vi "Test Buffer.vi"() -> ()   [LabVIEW 2017]
uses:
  PMU Buffer/Buffer state.ctl
  PMU Buffer/Buffer Settings.ctl
  PMU Buffer/Buffer DATA cluster.ctl
  PMU Buffer/PMU data buffer.lvlib
panel:
  out "Service 2 (All Buffer)":sgl[](array[numeric])
  out "Service 1 (Last 20)":sgl[](array[numeric])
  out "Should Get: 2":dbl[](array[numeric])
  out "Service 2 (1 shot)":sgl[](array[numeric])
  out "Service 1 (1 by 1)":sgl[](array[numeric])
  out "Should Get:":dbl[](array[numeric])
  # "Tests \nTest 1: Add and retrieve elements 1 by 1 in the buffer and fill the buffer entirely:\n- Compare the concatenated output of service 1 and the full output of service 2\nTest 2: Add 1 more element:\n- Compare the output of getting the whole buffer (Service 2) and the last <buffer size> elements (service 1)"
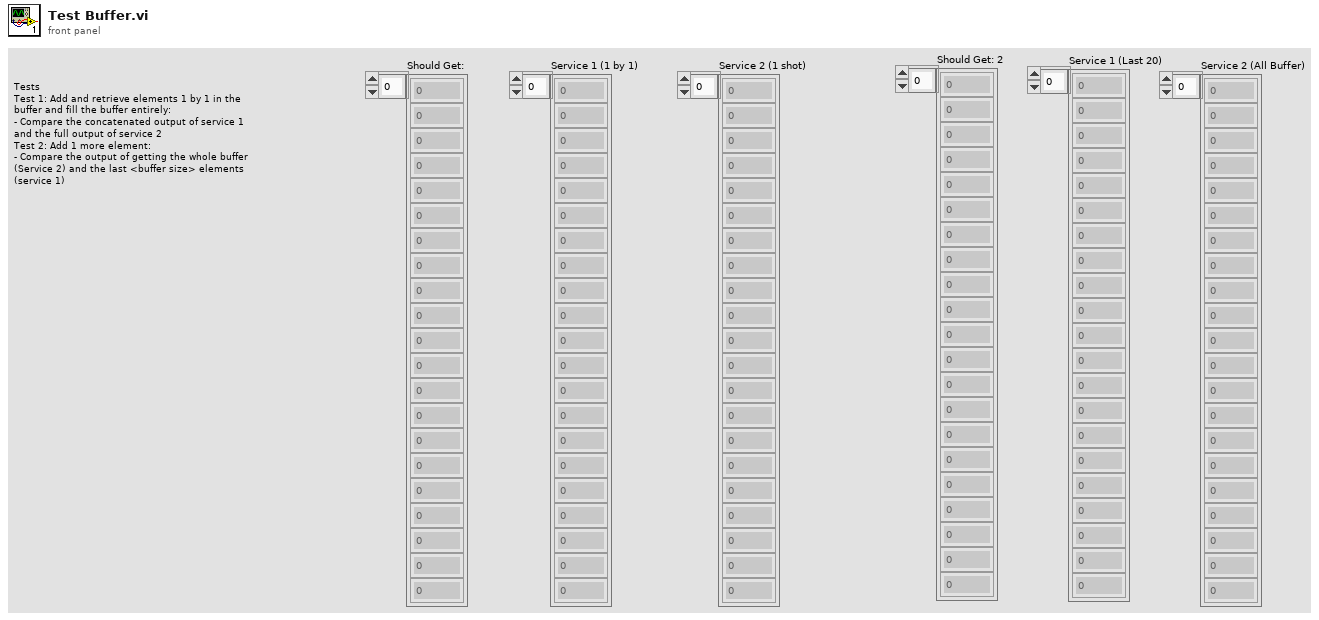
[diagram p1: front panel]
types:
  T1 = typedef "PMU data buffer.lvlib/Buffer DATA cluster.ctl" = cluster{timestamp, csg[], sgl[]}
  T2 = typedef "PMU data buffer.lvlib/Buffer state.ctl" = enum16{"Init", "Change Size", "Flush", "Exit", "Add", "Get", "Hist_Toggle", "Add_Serv"}
  T3 = typedef "PMU data buffer.lvlib/Buffer Settings.ctl" = cluster{"Index":i32, "Size":i32, "Samples":i32, "Ordered ?":bool}
  T4 = typedef "PMU data buffer.lvlib/Buffer DATA OUT ordered.ctl" = cluster{"Timestamp":timestamp[], "Phasor":csg[][], "Analog":sgl[][]}
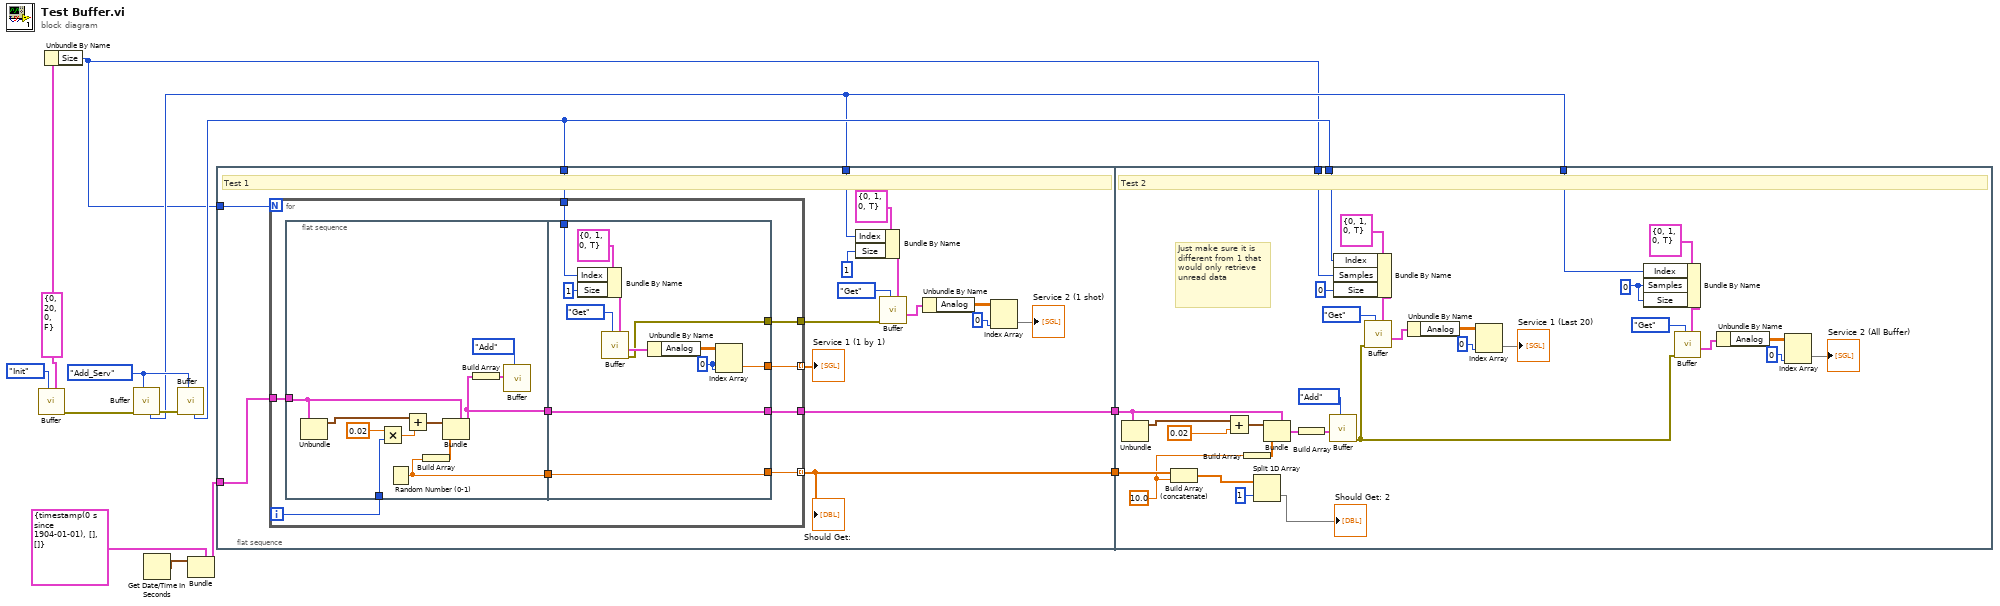
[diagram p0: block diagram]
diagram:
  w6 = Buffer_state."Add_Serv" ("Mode")
  w8 = T3 {"Index"=0, "Size"=20, "Samples"=0, "Ordered ?"=FALSE} ("Parameters")
  n1 = call "Buffer.vi"("Parameters"=w8, "Mode"=Buffer_state."Init") -> ("Error OUT"=w13:errorcluster)  [unwired: 5 in, 4 out]
  n2 = Unbundle By Name(w8) -> ("Size"=w1:i32)
  n3 = call "Buffer.vi"("Mode"=w6, "Error IN"=w13) -> ("Error OUT"=w7:errorcluster, "Index"=w2:i32)  [unwired: 5 in, 3 out]
  n4 = Get Date/Time In Seconds() -> (seconds since 1Jan1904=w9:timestamp)
  n5 = call "Buffer.vi"("Mode"=w6, "Error IN"=w7) -> ("Index"=w3:i32)  [unwired: 5 in, 4 out]
  n6 = Bundle(cluster=T1 {timestamp(0 s since 1904-01-01), [], []} ("PMU data buffer.lvlib:Buffer DATA cluster"), w9) -> (w10:T1)  [unwired: 2 in]
  n7 = flat-sequence {
    tunnel: w10 -> [w29]
    tunnel: w3 -> [w15]
    tunnel: w2 -> [w17]
    tunnel: [w19] -> w5
    tunnel: [w18] -> w4
    tunnel: w1 -> [w14]
    tunnel: w5 -> [w94]
    tunnel: w4 -> [w86]
    tunnel: w3 -> [w71]
    tunnel: w2 -> [w70]
    tunnel: w1 -> [w62]
    frame #0 {
      # "Test 1"
      n8 = for {
        N: w14 -> [_]
        tunnel: w29 -> [w38]
        tunnel: [w35] -> w19 mode=indexing
        tunnel: [w34] -> w28 mode=indexing
        tunnel: [w32] -> w18
        tunnel: [w31] -> w16
        tunnel: w15 -> [w30]
        i -> [w37]
        n9 = flat-sequence {
          tunnel: w38 -> [w47]
          tunnel: w37 -> [w43]
          tunnel: [w40] -> w36
          tunnel: [w39] -> w33
          tunnel: [w56] -> w35
          tunnel: w36 -> [w56]
          tunnel: [w53] -> w34
          tunnel: w33 -> [w52]
          tunnel: [w52] -> w32
          tunnel: [w51] -> w31
          tunnel: w30 -> [w50]
          frame #0 {
            n10 = Unbundle(w47) -> (w46:timestamp)  [unwired: 2 out]
            n11 = Multiply(x=0.02, y=w43) -> (x*y=w44:dbl)
            n12 = Random Number (0-1)() -> (number: 0 to 1=w40:dbl)
            n13 = Add(x=w46, y=w44) -> (x+y=w45:timestamp)
            n14 = Build Array(w40) -> (w41:dbl[])
            n15 = Bundle(cluster=w47, w45, w41) -> (w39:T1)  [unwired: 1 in]
            n16 = Build Array(w39) -> (w48:T1[])
            n17 = call "Buffer.vi"("Mode"=Buffer_state."Add", "DATA IN"=w48) -> ()  [unwired: 5 in, 5 out]
          }
          frame #1 {
            w54 = 0 ("index (row)")
            n18 = Bundle By Name(cluster=T3 {"Index"=0, "Size"=1, "Samples"=0, "Ordered ?"=TRUE} ("Parameters"), "Index"=w50, "Size"=1) -> (w59:T3)
            n19 = call "Buffer.vi"("Parameters"=w59, "Mode"=Buffer_state."Get") -> ("Error OUT"=w51:errorcluster, "Output"=w58:T4)  [unwired: 5 in, 3 out]
            n20 = Unbundle By Name(w58) -> ("Analog"=w55:sgl[][])
            n21 = Index Array(array=w55, index (row)=w54, index (col)=w54) -> (element=w53:sgl)
          }
        }
      }
      "Should Get:" <- w19
      "Service 1 (1 by 1)" <- w28
      n22 = Bundle By Name(cluster=T3 {"Index"=0, "Size"=1, "Samples"=0, "Ordered ?"=TRUE} ("Parameters"), "Index"=w17, "Size"=1) -> (w26:T3)
      n23 = call "Buffer.vi"("Parameters"=w26, "Mode"=Buffer_state."Get", "Error IN"=w16) -> ("Output"=w22:T4)  [unwired: 4 in, 4 out]
      n24 = Unbundle By Name(w22) -> ("Analog"=w23:sgl[][])
      n25 = Index Array(array=w23, index (col)=0 ("index (row)")) -> (element=→"Service 2 (1 shot)":sgl[])  [unwired: 1 in]
    }
    frame #1 {
      w63 = 0 ("Size")
      w90 = 10.0 ("number: 0 to 1")
      # "Just make sure it is different from 1 that would only retrieve unread data"
      # "Test 2"
      n26 = Unbundle(w86) -> (w91:timestamp)  [unwired: 2 out]
      n27 = Build Array (concatenate)(w94, w90) -> (w68:dbl[])
      n28 = Add(x=w91, y=0.02 ("x")) -> (x+y=w92:timestamp)
      n29 = Build Array(w90) -> (w93:dbl[])
      n30 = Split 1D Array(array=w68, index=1) -> (second subarray=→"Should Get: 2":dbl[])  [unwired: 1 out]
      n31 = Bundle(cluster=w86, w92, w93) -> (w87:T1)  [unwired: 1 in]
      n32 = Build Array(w87) -> (w89:T1[])
      n33 = call "Buffer.vi"("Mode"=Buffer_state."Add", "DATA IN"=w89) -> ("Error OUT"=w69:errorcluster)  [unwired: 5 in, 4 out]
      n34 = Bundle By Name(cluster=T3 {"Index"=0, "Size"=1, "Samples"=0, "Ordered ?"=TRUE} ("Parameters"), "Index"=w71, "Samples"=w62, "Size"=0) -> (w79:T3)
      n35 = call "Buffer.vi"("Parameters"=w79, "Mode"=Buffer_state."Get", "Error IN"=w69) -> ("Output"=w83:T4)  [unwired: 4 in, 4 out]
      n36 = Unbundle By Name(w83) -> ("Analog"=w82:sgl[][])
      n37 = Index Array(array=w82, index (col)=0 ("index (row)")) -> (element=→"Service 1 (Last 20)":sgl[])  [unwired: 1 in]
      n38 = Bundle By Name(cluster=T3 {"Index"=0, "Size"=1, "Samples"=0, "Ordered ?"=TRUE} ("Parameters"), "Index"=w70, "Samples"=w63, "Size"=w63) -> (w78:T3)
      n39 = call "Buffer.vi"("Parameters"=w78, "Mode"=Buffer_state."Get", "Error IN"=w69) -> ("Output"=w74:T4)  [unwired: 4 in, 4 out]
      n40 = Unbundle By Name(w74) -> ("Analog"=w75:sgl[][])
      n41 = Index Array(array=w75, index (col)=0 ("index (row)")) -> (element=→"Service 2 (All Buffer)":sgl[])  [unwired: 1 in]
    }
  }
